vi "Element Init.vi"(7 "VolatusAPI":refnum<class "VolatusAPI.lvclass">, 8 "error in (no error)":errorcluster, 10 "JSON":string, 11 "DblPopupControl in":refnum<class "DblPopupControl.lvclass">) -> (0 "error out":errorcluster, 3 "DblPopupControl out":refnum<class "DblPopupControl.lvclass">)   [LabVIEW 2020, in "VolatusGUIElements.lvlib" / "DblPopupControl.lvclass"]
uses:
  DblPopupControl.lvclass
  C:/dev/lv20CE/relink/lv-volatus/VolatusGUI/GUI Element/GUI Element.lvclass
  Volatus/VolatusAPI/VolatusAPI.lvclass
  JSON.ctl
  lv-vecto/Vecto/Group DBL/Group DBL.lvclass
  C:/dev/lv20CE/relink/lv-vecto/Vecto/Group/Group.lvclass
  Cmd State.ctl
  VolatusGUI/GUI Element/GUI Element.lvclass/GUI Element.ctl
  DblPopupControl.lvclass/DblPopupControl.ctl
  9743c59a-7e7e-4945-bb31-9bc961dfa8ed.vi
  <vilib>/JDP Science/JSONtext/JSON text to Variant.vi
  <vilib>/JDP Science/JSONtext/LVClass Serializer/JSONtext LVClass Serializer.lvclass
  VolatusGUI/GUI Element/GUI Element.lvclass
  VolatusGUI/Element Inhibit/Element Inhibit.lvclass
  Volatus/Numeric Command/Numeric Command.lvclass
  C:/dev/lv20CE/relink/lv-volatus/VolatusGUIElements/DblPopupControl/DblPopupControl.lvclass
  C:/dev/lv20CE/relink/lv-volatus/VolatusGUI/OnMouseDown/OnMouseDown.lvclass
  C:/dev/lv20CE/relink/lv-vecto/Vecto/Group DBL/Group DBL.lvclass
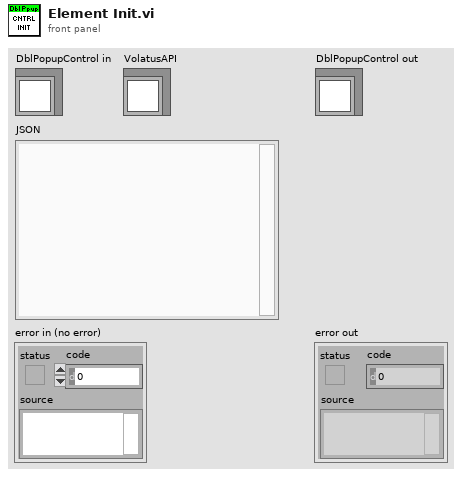
[diagram p1: front panel]
types:
  T1 = typedef "VolatusGUIElements.lvlib/DblPopupControl.lvclass/Cmd State.ctl" = cluster{"Commanding":bool, "Start":dbl, "Error":bool, "Value":dbl}
  T2 = typedef "VolatusGUIElements.lvlib/DblPopupControl.lvclass/JSON.ctl" = cluster{"Channel":string, "Format":string, "Staleness":dbl, "Inhibit":string}
  T3 = typedef "VectoConfig.lvlib/Channel Info.ctl" = cluster{"Name":string, "Group":string, "Owning Node":string, "Owning Task":string, "Resource":string}
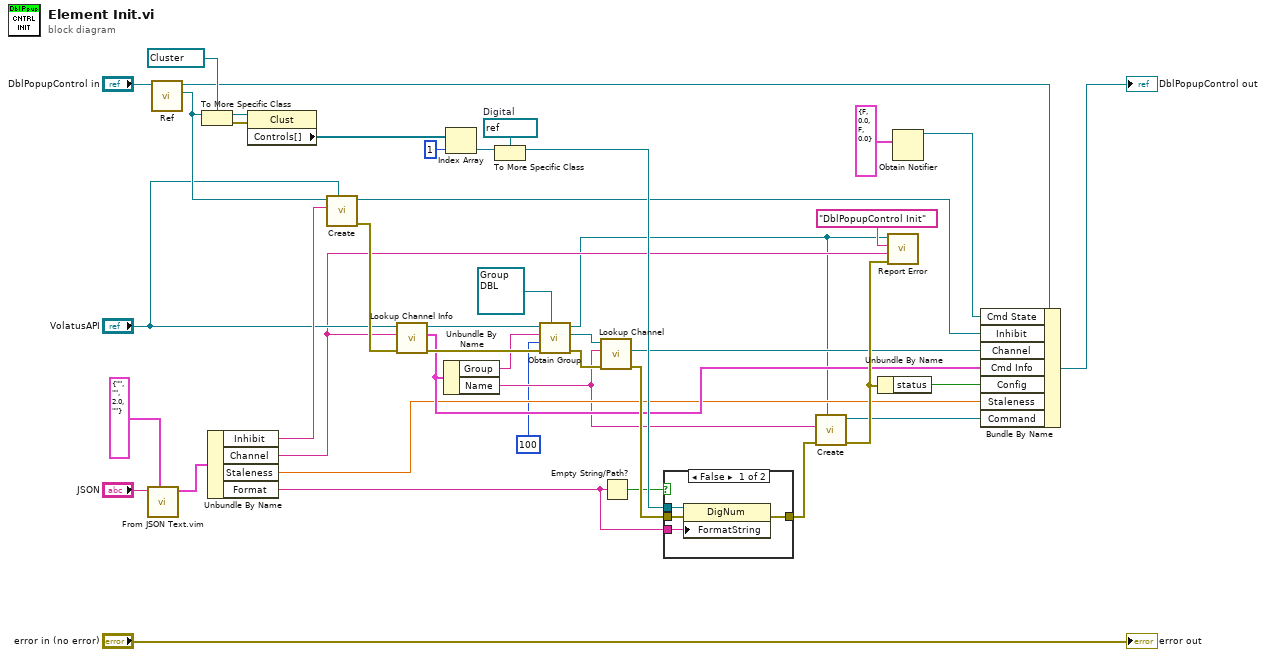
[diagram p0: block diagram]
diagram:
  w33 = refnum<vi> refnum  # Digital
  n1 = call "From JSON Text.vim"("Data Type and Default Value"=T2 {"Channel"="", "Format"="", "Staleness"=2.0, "Inhibit"=""} ("JSON"), "JSON"="JSON") -> ("Data out"=w37:T2)  [unwired: 8 in, 1 out]
  n2 = call "Ref.vi"("GUI Element in"="DblPopupControl in") -> ("Ref"=w10:refnum<vi>, "GUI Element out"=w21:refnum<class "DblPopupControl.lvclass">)  [unwired: 9 in]
  n3 = To More Specific Class(target class=refnum<vi> refnum ("specific class reference"), reference=w10) -> (specific class reference=w35:refnum<vi>, error out=w34:errorcluster)  [unwired: 1 in]
  n4 = Unbundle By Name(w37) -> ("Inhibit"=w11:string, "Channel"=w4:string, "Staleness"=w14:dbl, "Format"=w12:string)
  n5 = property class="Clust"(reference=w35, error in=w34) -> ("Controls[]"=w32:refnum<vi>[])  [unwired: 2 out]
  n6 = call "Create.vi"("VolatusAPI"="VolatusAPI", "Inhibit Channel"=w11, "Control Ref"=w10) -> ("error out"=w42:errorcluster, "Element Inhibit out"=w8:refnum<class "Element Inhibit.lvclass">)  [unwired: 7 in]
  n7 = call "Lookup Channel Info.vi"("error in (no error)"=w42, "Channel Name"=w4, "VolatusAPI in"="VolatusAPI") -> ("error out"=w24:errorcluster, "Channel Info"=w19:T3, "VolatusAPI out"=w23:refnum<class "VolatusAPI.lvclass">)  [unwired: 5 in, 1 out]
  n8 = Unbundle By Name(w19) -> ("Group"=w22:string, "Name"=w7:string)
  n9 = Index Array(array=w32, index=1) -> (element=w30:refnum<vi>)
  n10 = To More Specific Class(target class=w33, reference=w30) -> (specific class reference=w28:refnum<vi>)  [unwired: 1 in, 1 out]
  n11 = call "Obtain Group.vi"("Group Type (Abstract)"=refnum<class "Group DBL.lvclass"> refnum ("Vecto.lvlib:Group.lvclass"), "error in (no error)"=w24, "Timeout ms (5000)"=u32 100, "Group Name"=w22, "VolatusAPI in"=w23) -> ("error out"=w25:errorcluster, "Group"=w26:refnum<class "Group DBL.lvclass">, "VolatusAPI out"=w2:refnum<class "VolatusAPI.lvclass">)  [unwired: 4 in]
  n12 = call "Lookup Channel.vi"("error in (no error)"=w25, "Channel Name"=w7, "Group in"=w26) -> ("error out"=w41:errorcluster, "Channel"=w20:refnum<class "Channel DBL.lvclass">)  [unwired: 6 in, 1 out]
  n13 = Empty String/Path?(string/path=w12) -> (empty?=w13:bool)
  n14 = case shown="False" w13 {
    tunnel: w41 -> [w47 w48]
    tunnel: w28 -> [w46 _]
    tunnel: w12 -> [w45 _]
    tunnel: [w44 w48] -> w3
    frame False {
      n15 = property class="DigNum"(reference=w46, error in=w47, "FormatString"=w45) -> (error out=w44:errorcluster)  [unwired: 1 out]
    }
    frame True {
    }
  }
  n16 = call "Create.vi"("VolatusAPI"=w2, "error in (no error)"=w3, "Channel"=w7) -> ("error out"=w43:errorcluster, "Numeric Command out"=w6:refnum<class "Numeric Command.lvclass">)  [unwired: 7 in]
  n17 = Unbundle By Name(w43) -> ("status"=w18:bool)
  n18 = call "Report Error.vi"("error in (no error)"=w43, "Message"=w4, "Context"="DblPopupControl Init", "VolatusAPI in"=w2) -> ()  [unwired: 6 in, 2 out]
  n19 = Obtain Notifier(notification data type=T1 {"Commanding"=FALSE, "Start"=0.0, "Error"=FALSE, "Value"=0.0} ("Cmd State")) -> (notifier out=w15:refnum<notifier>)  [unwired: 3 in, 2 out]
  n20 = Bundle By Name(cluster=w21, "Cmd State"=w15, "Inhibit"=w8, "Channel"=w20, "Cmd Info"=w19, "Config"=w18, "Staleness"=w14, "Command"=w6) -> (→"DblPopupControl out":refnum<class "DblPopupControl.lvclass">)
  "error out" <- "error in (no error)"
